vi "StateMachineLogger.vi"(0 "reference in":refnum<class "Logger.lvclass">, 5 "error in (no error)":errorcluster, 9 "SV_Publisher in":refnum<class "SV_Publisher.lvclass">) -> ()   [LabVIEW 2019, in "Logger.lvclass"]
uses:
  Logger.lvclass
  State.ctl
  EventData.ctl
  EventType.ctl
  TypeDef/AlarmType.ctl
  SV_Puplisher_class/SV_Publisher.lvclass
  Logger.lvclass/Logger.ctl
  DatabaseInterface_class/DatabaseInterface.lvclass
panel:
  out "All Events":set{T1}(c389)
  out "Table Events":string[][](table)
  out "Table Objects":string[][](table)
  out "State":T4
  out "error handle":errorcluster
  out "error connect":errorcluster
  out "error initiate":errorcluster
  out "error disconnect":errorcluster
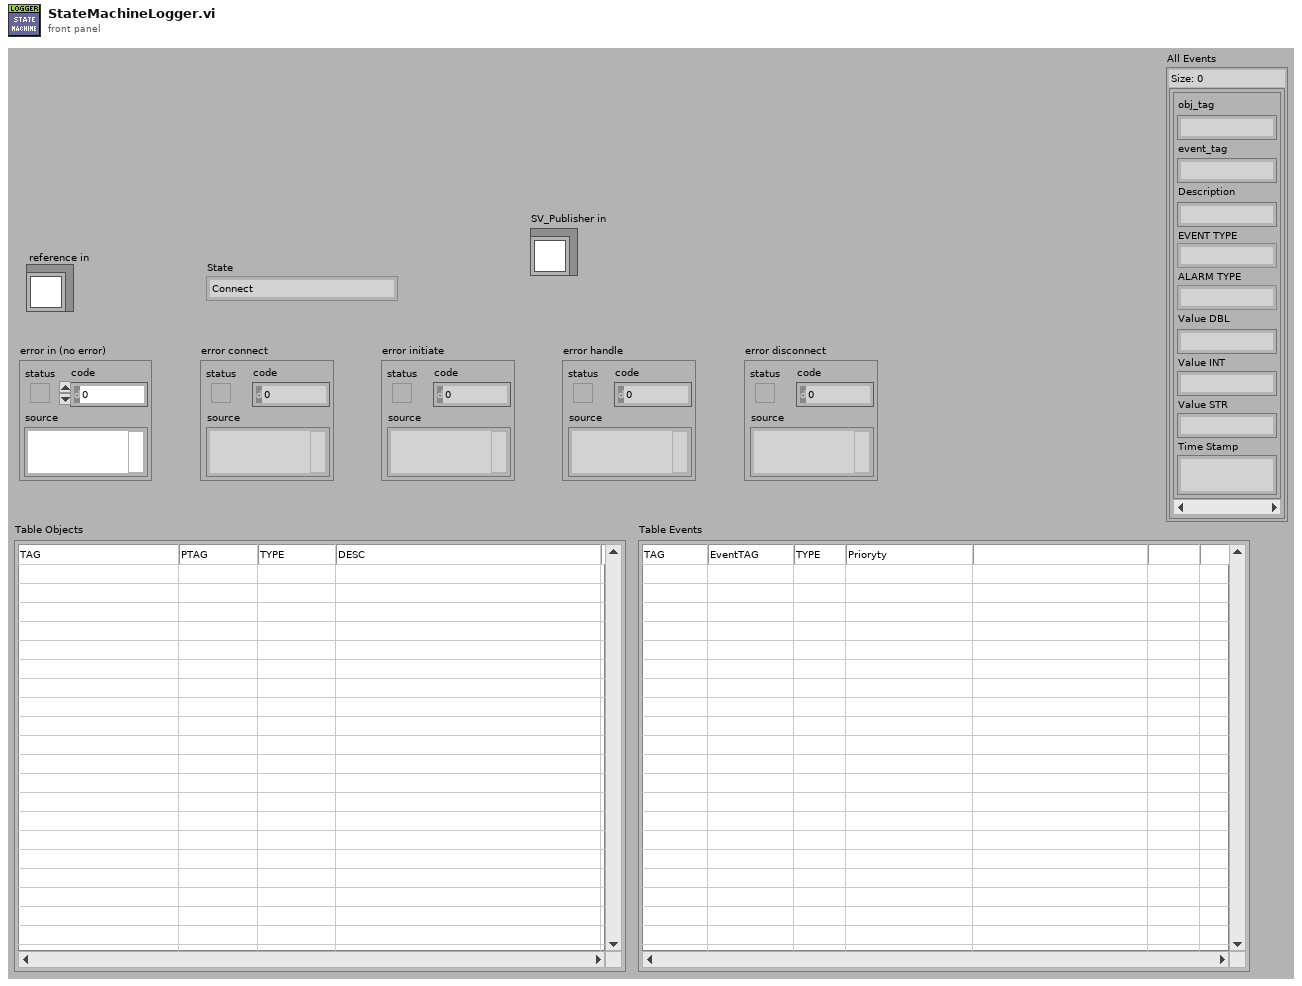
[diagram p1: front panel]
types:
  T1 = typedef "Logger.lvclass/EventData.ctl" = cluster{"obj_tag":string, "event_tag":string, "Description":string, "EVENT TYPE":T2, "ALARM TYPE":T3, "Value DBL":dbl, "Value INT":i32, "Value STR":string, "Time Stamp":timestamp}
  T2 = typedef "Logger.lvclass/EventType.ctl" = enum16{"DI_LO", "DI_HI", "DO_LO", "DO_HI", "DA_LO", "DA_HI", "AA_LO", "AA_HI", "CMD", "ERR", "ST"}
  T3 = typedef "AlarmType.ctl" = enum16{"Normal", "Warning", "Alarm"}
  T4 = typedef "Logger.lvclass/State.ctl" = enum16{"Connect", "Initiate", "Handle", "Disconect"}
  T5 = typedef "Logger.lvclass/ObjData.ctl" = cluster{"object_tag":string, "parent_tag":string, "object_type":T6, "description":string}
  T6 = typedef "Logger.lvclass/ObjType.ctl" = enum16{"Procces", "Device", "Signal", "DI", "DO", "DA", "AI", "AO", "AA"}
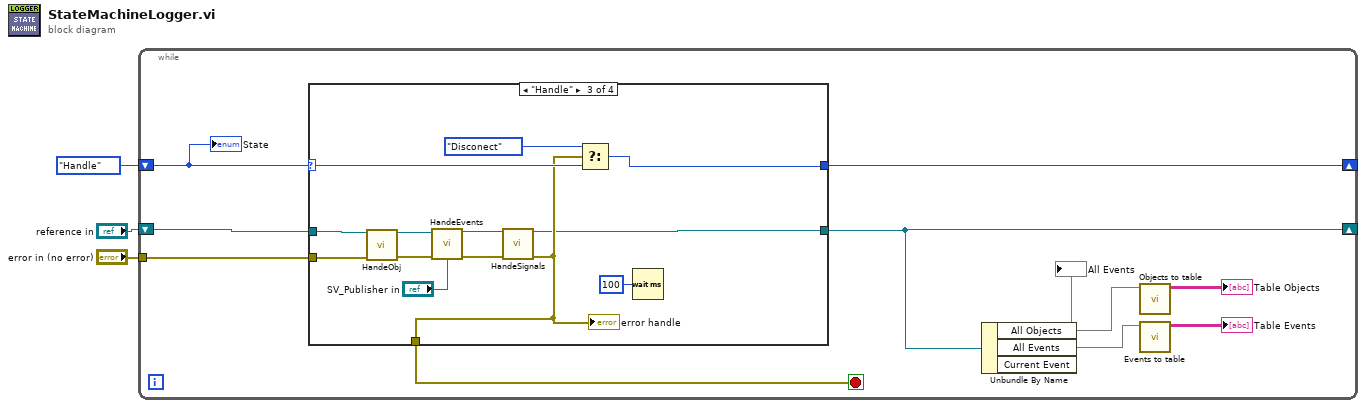
[diagram p0: block diagram]
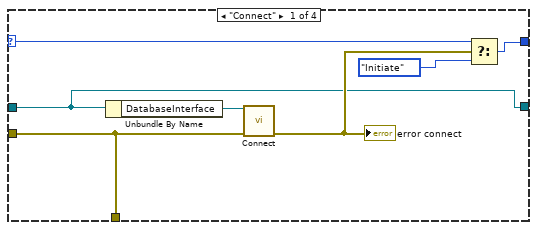
[diagram p2: hidden frame]
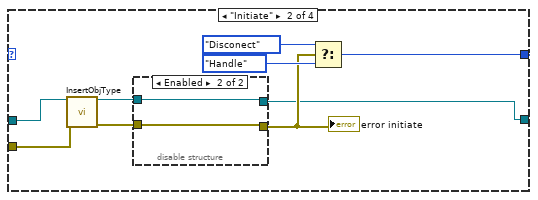
[diagram p3: hidden frame]
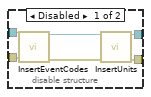
[diagram p4: hidden frame]
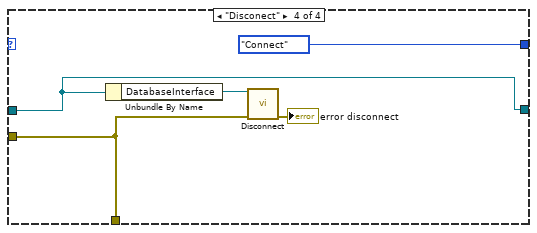
[diagram p5: hidden frame]
diagram:
  n1 = while {
    tunnel: "error in (no error)" -> [w11]
    shift-right: [w10] -> _
    shift-left: State."Handle" ("State") -> [w13]
    shift-right: [w8] -> _
    shift-left: "reference in" -> [w12]
    stop <- w9 stop-if-true
    n2 = case shown="\"Handle\"" w13 {
      selector: w13 -> [w18 _ w44 _]
      tunnel: w12 -> [w14 w29 w50 w51]
      tunnel: w11 -> [w20 w28 w49 w55]
      tunnel: [w16 w23 w42 State."Connect" ("State")] -> w10
      tunnel: [w20 _ w40 w55] -> w9
      tunnel: [w14 w21 w39 w51] -> w8
      frame "Connect" {
        n3 = Unbundle By Name(w14) -> ("DatabaseInterface"=w19:refnum<class "DatabaseInterface.lvclass">)
        n4 = call-dynamic "Connect.vi"("reference in"=w19, "error in (no error)"=w20) -> ("error out"=w15:errorcluster)  [unwired: 12 in, 1 out]
        "error connect" <- w15
        n5 = Select(t=w18, s=w15, f=State."Initiate") -> (s? t:f=w16:T4)
      }
      frame "Initiate" {
        n6 = call "InsertObjType.vi"("reference in"=w29, "error in (no error)"=w28) -> ("reference out"=w27:refnum<class "Logger.lvclass">, "error out"=w26:errorcluster)  [unwired: 11 in, 1 out]
        n7 = disable-structure shown="Enabled" {
          disable-tunnel: w27 -> [w35 w37]
          disable-tunnel: w26 -> [w34 w36]
          disable-tunnel: [w31 w36] -> w22
          disable-tunnel: [w30 w37] -> w21
          frame Disabled {
            n8 = call "InsertEventCodes.vi"("reference in"=w35, "error in (no error)"=w34) -> ("reference out"=w33:refnum<class "Logger.lvclass">, "error out"=w32:errorcluster)  [unwired: 11 in, 1 out]
            n9 = call "InsertUnits.vi"("reference in"=w33, "error in (no error)"=w32) -> ("reference out"=w30:refnum<class "Logger.lvclass">, "error out"=w31:errorcluster)  [unwired: 11 in, 1 out]
          }
          frame Enabled {
          }
        }
        "error initiate" <- w22
        n10 = Select(t=State."Disconect", s=w22, f=State."Handle") -> (s? t:f=w23:T4)
      }
      frame "Handle" {
        n11 = call "HandeObj.vi"("reference in"=w50, "error in (no error)"=w49) -> ("reference out"=w48:refnum<class "Logger.lvclass">, "error out"=w47:errorcluster)  [unwired: 10 in, 2 out]
        n12 = call "HandeEvents.vi"("reference in"=w48, "error in (no error)"=w47, "SV_Publisher in"="SV_Publisher in") -> ("reference out"=w45:refnum<class "Logger.lvclass">, "error out"=w46:errorcluster)  [unwired: 10 in, 1 out]
        n13 = call "HandeSignals.vi"("reference in"=w45, "error in (no error)"=w46) -> ("reference out"=w39:refnum<class "Logger.lvclass">, "error out"=w40:errorcluster)  [unwired: 11 in, 1 out]
        "error handle" <- w40
        n14 = Select(t=State."Disconect", s=w40, f=w44) -> (s? t:f=w42:T4)
        n15 = Wait (ms)(milliseconds to wait=u32 100) -> ()  [unwired: 1 out]
      }
      frame "Disconect" {
        n16 = Unbundle By Name(w51) -> ("DatabaseInterface"=w53:refnum<class "DatabaseInterface.lvclass">)
        n17 = call-dynamic "Disconnect.vi"("reference in"=w53, "error in (no error)"=w55) -> ("error out"=→"error disconnect":errorcluster)  [unwired: 12 in, 1 out]
      }
    }
    n18 = Unbundle By Name(w8) -> ("All Objects"=w7:set{T5}, "All Events"=w5:set{T1})  [unwired: 1 out]
    "All Events" <- w5
    n19 = call "Objects to table.vi"("All Objects"=w7) -> ("Table Control"=→"Table Objects":string[][])  [unwired: 9 in, 1 out]
    n20 = call "Events to table.vi"("All Events"=w5) -> ("Table Control"=→"Table Events":string[][])  [unwired: 9 in, 1 out]
    "State" <- w13
  }
